vi "Read_ini_Str.vi"(8 "error in (no error)":errorcluster, 9 "key":string, 10 "section":string, 11 "configuration file path":path) -> (0 "error out":errorcluster, 2 "value":string)   [LabVIEW 2015]
uses:
  <vilib>/Utility/config.llb/Read Key (String).vi
  <vilib>/Utility/config.llb/NI_LVConfig.lvlib
panel:
  out "found?":bool
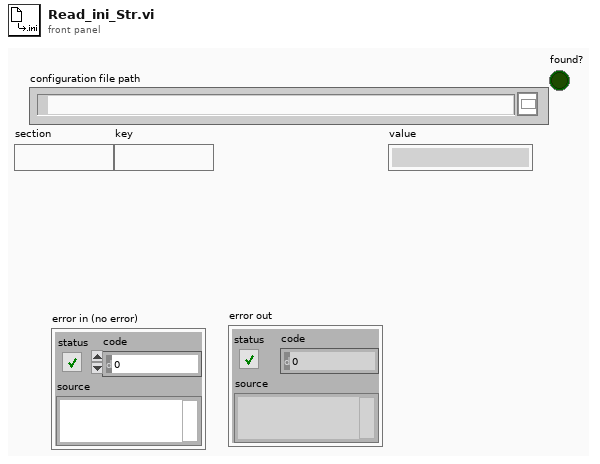
[diagram p1: front panel]
types:
  T1 = typedef "NI_LVConfig.lvlib/Config Data RefNum.ctl" = refnum<k1>
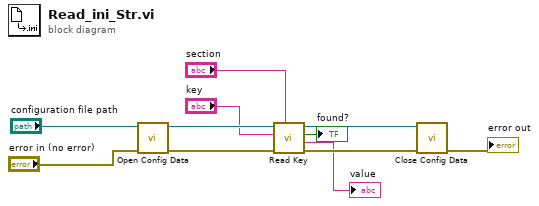
[diagram p0: block diagram]
diagram:
  n1 = call <vilib>:"Open Config Data.vi"("error in (no error)"="error in (no error)", "configuration file path"="configuration file path") -> ("error out"=w5:errorcluster, "refnum"=w6:T1)  [unwired: 7 in, 1 out]
  n2 = call-poly <vilib>:"Read Key.vi"("section"="section", "error in (no error)"=w5, "key"="key", "refnum"=w6) -> ("error out"=w10:errorcluster, "value"=→"value":string, "found?"=→"found?":bool, "refnum out"=w9:T1)  [unwired: 4 in]
  n3 = call <vilib>:"Close Config Data.vi"("error in (no error)"=w10, "refnum"=w9) -> ("error out"=→"error out":errorcluster)  [unwired: 8 in, 1 out]
